vi "Front Panel.vi"(11 "GUI In":refnum<class "CRD HK.lvclass">) -> ()   [LabVIEW 2015, in "CRD HK.lvclass"]
uses:
  CRD HK.lvclass
  Reusable/Xctls/Buffer/2D Control/2D Buffer Display.xctl
  Reusable/GUI/GUI.lvclass/GUI.ctl
  Reusable/Observer/Observer.lvclass/Observer.ctl
  CRDS/Data/cCRDS Data.lvclass
  Reusable/GUI/Accessors/Read RegEvent.vi
  Reusable/Observer/Read Data Queue.vi
  Reusable/CRDS/Data/Main/Read CellData.vi
  CRDS/Data/Read Humidifier T.vi
  Reusable/Data/Read measTime.vi
  Reusable/CRDS/Data/Cell/Read hkParam.vi
  Reusable/Data/Data.lvclass
  Reusable/CRDS/Data/Cell/CRDS Cell Data.lvclass
panel:
  out "crdHK":cluster{"data_out":sgl[][], "time":timestamp}(xcontrol)
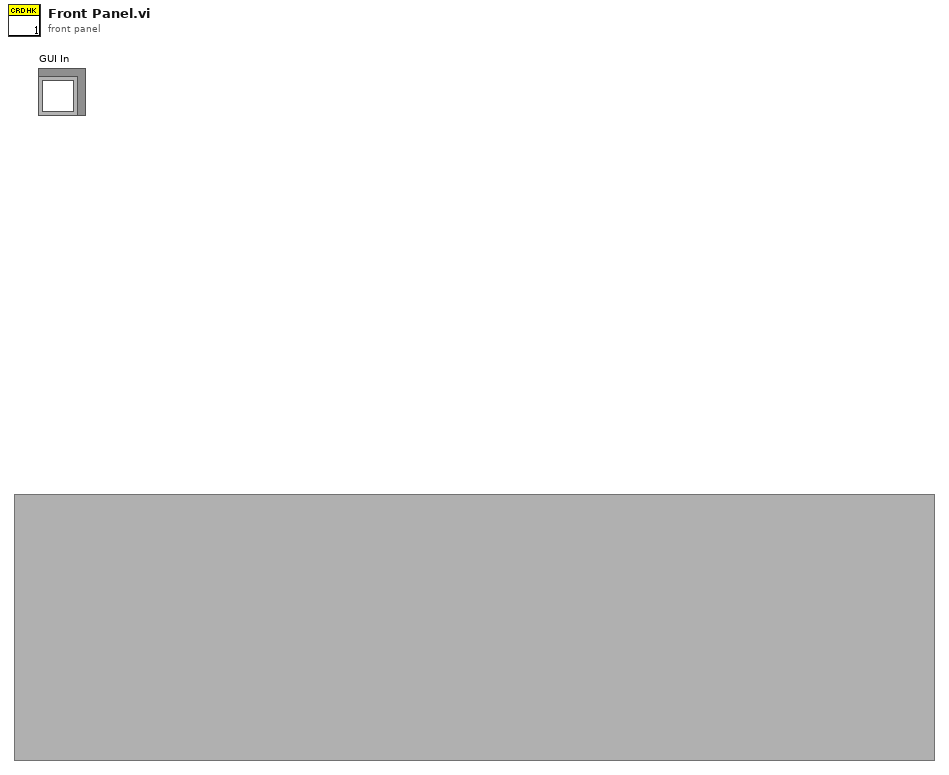
[diagram p1: front panel]
types:
  T1 = cluster{"Name":string, "Line Width":u8, "Line Style":u8, "Color":u32}[]
  T2 = typedef "calData.ctl" = cluster{"rhDilFac":sgl, "Q":sgl, "Tmean":sgl, "extDilFac":sgl, "rhCell":sgl, "P":sgl, "T":sgl}
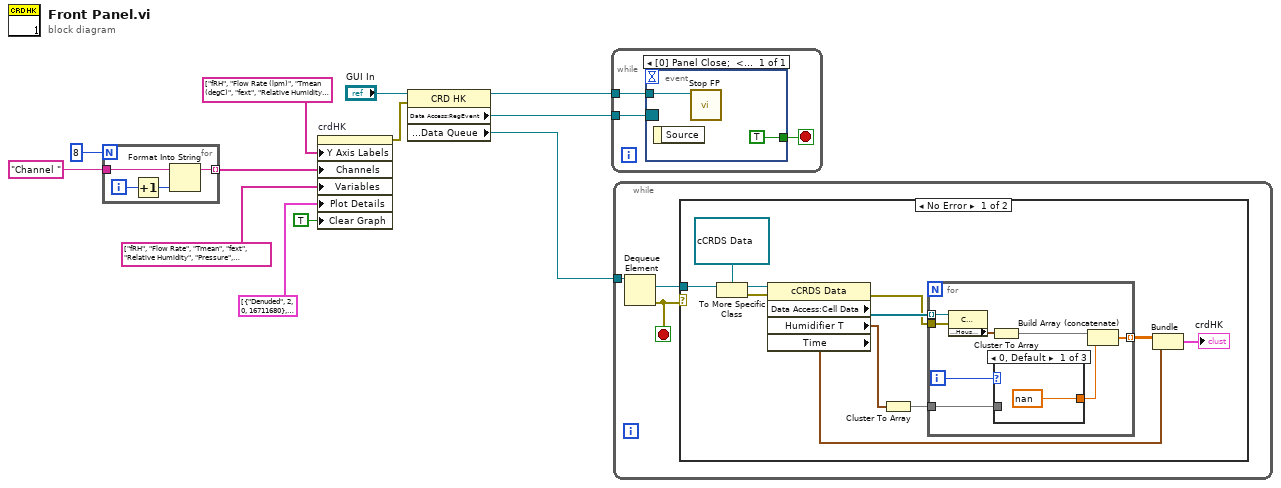
[diagram p0: block diagram]
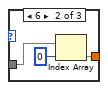
[diagram p2: hidden frame]
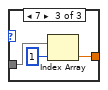
[diagram p3: hidden frame]
diagram:
  n1 = for {
    N: 8 -> [_]
    tunnel: "Channel " -> [w14]
    tunnel: [w13] -> w4 mode=indexing
    i -> [w16]
    n2 = Increment(x=w16) -> (x+1=w15:i32)
    n3 = Format Into String(initial string=w14, w15) -> (resulting string=w13:string)  [unwired: 2 in, 1 out]
  }
  n4 = property on="crdHK" class="2D Buffer Display (strict)"("Y Axis Labels"=string[] ["fRH", "Flow Rate (lpm)", "Tmean (degC)", "fext", "Relative Humidity (%)", "Pressure (mb)", "Temperature (degC)", "Saturator Temperature (degC)"], "Channels"=w4, "Variables"=string[] ["fRH", "Flow Rate", "Tmean", "fext", "Relative Humidity", "Pressure", "Temperature", "Saturator Temperature"], "Plot Details"=T1 [{"Name"="Denuded", "Line Width"=2, "Line Style"=0, "Color"=16711680}, {"Name"="Denuded", "Line Width"=2, "Line Style"=1, "Color"=16860}, {"Name"="Gas", "Line Width"=2, "Line Style"=0, "Color"=33023}, {"Name"="Dry", "Line Width"=2, "Line Style"=0, "Color"=16512}, {"Name"="Dry", "Line Width"=2, "Line Style"=0, "Color"=8388672}, {"Name"="Dry", "Line Width"=2, "Line Style"=1, "Color"=6618880}, {"Name"="Med RH", "Line Width"=2, "Line Style"=1, "Color"=1985280}, {"Name"="High RH", "Line Width"=2, "Line Style"=1, "Color"=32832}], "Clear Graph"=TRUE) -> (error out=w2:errorcluster)  [unwired: 2 in, 1 out]
  n5 = property class="CRD HK"(reference="GUI In", error in=w2) -> (reference out=w1:refnum<class "CRD HK.lvclass">, "Data Access:RegEvent"=w12:refnum<event-registration>, "Data Access:Data Queue"=w11:refnum<queue>)  [unwired: 1 out]
  n6 = while {
    tunnel: w12 -> [w18]
    tunnel: w1 -> [w17]
    stop <- w19 stop-if-true
    n7 = event shown="[0] Panel Close;  <True>: User Event" {
      selector: w18 -> [_]
      dyn-events: _ -> [_]
      timeout: _ -> [_]
      tunnel: [TRUE] -> w19
      tunnel: w17 -> [w20]
      event Panel Close; User Event {
        n8 = event-data() -> ()  [unwired: 1 in, 1 out]
        n9 = call-dynamic "Stop FP.vi"("GUI in"=w20) -> ()  [unwired: 9 in, 2 out]
      }
    }
  }
  n10 = while {
    tunnel: w11 -> [w24]
    stop <- w23 stop-if-true
    n11 = Dequeue Element(queue=w24) -> (element=w22:refnum<data-value>, error out=w23:errorcluster)  [unwired: 2 in, 2 out]
    n12 = case shown="No Error" w23 {
      tunnel: w22 -> [w33 _]
      frame No Error {
        n13 = To More Specific Class(target class=refnum<data-value> refnum ("data value reference"), reference=w33) -> (specific class reference=w32:refnum<data-value>, error out=w29:errorcluster)  [unwired: 1 in]
        n14 = property class="cCRDS Data"(reference=w32, error in=w29) -> (error out=w34:errorcluster, "Data Access:Cell Data"=w35:refnum<class "CRDS Cell Data.lvclass">[], "Humidifier T"=w26:cluster{"Hum 1":sgl, "Hum 2":sgl}, "Time"=w27:timestamp)  [unwired: 1 out]
        n15 = Cluster To Array(cluster=w26) -> (array=w25:sgl[])
        n16 = for {
          tunnel: w35 -> [w43] mode=indexing
          tunnel: w34 -> [w42]
          tunnel: [w37] -> w30 mode=indexing
          tunnel: w25 -> [w39]
          i -> [w40]
          n17 = property class="CRDS Cell"(reference=w43, error in=w42) -> ("Data Access:Housekeeping"=w41:T2)  [unwired: 2 out]
          n18 = Cluster To Array(cluster=w41) -> (array=w36:sgl[])
          n19 = case shown="0, Default" w40 {
            tunnel: [sgl nan w45 w48] -> w38
            tunnel: w39 -> [_ w46 w49]
            frame 0, Default {
            }
            frame 6 {
              n20 = Index Array(array=w46, index=0) -> (element=w45:sgl)
            }
            frame 7 {
              n21 = Index Array(array=w49, index=1) -> (element=w48:sgl)
            }
          }
          n22 = Build Array (concatenate)(w36, w38) -> (w37:sgl[])
        }
        n23 = Bundle(w30, "Time"=w27) -> (→"crdHK":cluster{sgl[][], "Time":timestamp})  [unwired: 1 in]
      }
      frame Error {
      }
    }
  }
